vi "MissingInProject.vi"(8 "error in":errorcluster, 11 "File Path":path) -> (0 "error out":errorcluster, 1 "Missing Files":string, 2 "Passed":bool)   [LabVIEW 2020, in "Missing in Project Tests.lvlib"]
uses:
  Missing in Project Tests.lvlib
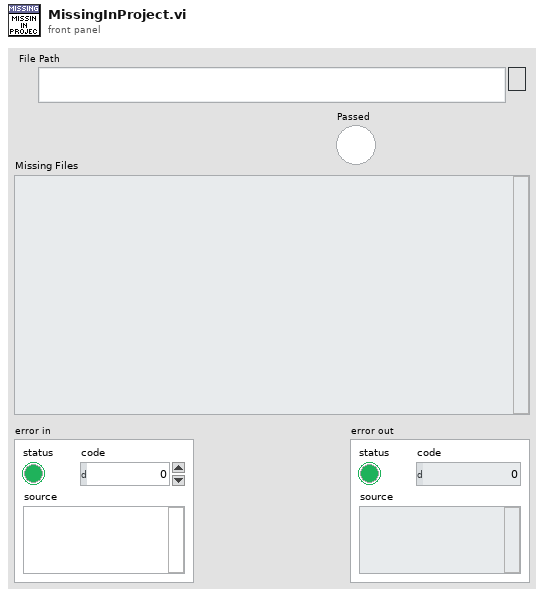
[diagram p1: front panel]
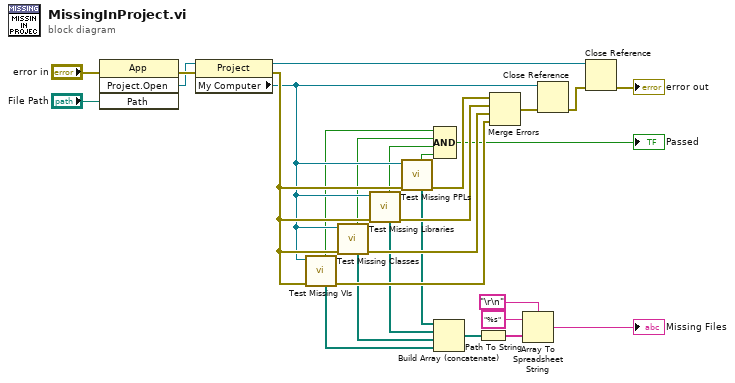
[diagram p0: block diagram]
diagram:
  n1 = invoke class="App" method="Project.Open"(error in="error in", "Path"="File Path") -> (error out=w28:errorcluster, "Project:Open"=w19:refnum<vi>)  [unwired: 2 in, 2 out]
  n2 = property class="Project"(reference=w19, error in=w28) -> (reference out=w17:refnum<vi>, error out=w20:errorcluster, "My Computer"=w16:refnum<vi>)
  n3 = call "Test Missing VIs.vi"("error in"=w20, "My Computer"=w16) -> ("error out"=w23:errorcluster, "Missing items"=w7:path[], "Pass"=w11:bool)  [unwired: 7 in]
  n4 = call "Test Missing Classes.vi"("error in"=w20, "My Computer"=w16) -> ("error out"=w24:errorcluster, "Missing items from LabVIEW project"=w8:path[], "Pass"=w12:bool)  [unwired: 7 in]
  n5 = call "Test Missing Libraries.vi"("error in"=w20, "My Computer"=w16) -> ("error out"=w25:errorcluster, "Missing items from LabVIEW project"=w9:path[], "Pass"=w13:bool)  [unwired: 7 in]
  n6 = call "Test Missing PPLs.vi"("error in"=w20, "My Computer"=w16) -> ("error out"=w26:errorcluster, "Missing items from LabVIEW project"=w10:path[], "Pass"=w14:bool)  [unwired: 7 in]
  n7 = Compound Arithmetic op=AND(w11, w12, w13, w14) -> (→"Passed":bool)
  n8 = Build Array (concatenate)(w10, w9, w8, w7) -> (w6:path[])
  n9 = Path To String(path=w6) -> (string=w5:string[])
  n10 = Merge Errors(w26, w25, w24, w23) -> (w22:errorcluster)
  n11 = Array To Spreadsheet String(delimiter (Tab)="\r\n", array=w5, 3:"%s" ("format string")) -> (spreadsheet string=→"Missing Files":string)
  n12 = Close Reference(reference=w16, error in (no error)=w22) -> (error out=w27:errorcluster)
  n13 = Close Reference(reference=w17, error in (no error)=w27) -> (error out=→"error out":errorcluster)
